vi "read_db_for_file_relocation.vi"(7 "Small?":bool, 8 "error in (no error)":errorcluster, 11 "File Location":T1=-2 items=["Unknown"=-5, "IDL Processing"=-4, "Writing from Queue"=-3, "Labview Files"=-2, "Retry Labview files"=-1, "Local Cache "=0, "Storage"=1]) -> (0 "error out":errorcluster, 3 "BP Array":T2[](array[typedef]) {"File Location" items=["Unknown"=-5, "IDL Processing"=-4, "Writing from Queue"=-3, "Labview Files"=-2, "Retry Labview files"=-1, "Local Cache "=0, "Storage"=1]})   [LabVIEW 2013]
uses:
  Batch Processor/bp_cluster.ctl
  Controls/File_location.ctl
  <vilib>/addons/database/Auxilliary.llb/DB Tools Parameter Info.ctl
  <vilib>/addons/database/Auxilliary.llb/DB Tools DataTypes.ctl
  <vilib>/addons/database/Auxilliary.llb/DB Tools Parameter Dir.ctl
  <vilib>/addons/database/Command.llb/Cmd Set Parameter Value (C).vi
  <vilib>/addons/database/Command.llb/Cmd Execute.vi
  <vilib>/addons/database/Recordset.llb/Rec Fetch Recordset Data (CR).vi
  <vilib>/addons/database/Recordset.llb/Rec Destroy - Command.vi
  <vilib>/addons/database/Command.llb/Cmd Delete.vi
  <vilib>/addons/database/_DB Variant To Data/Database Variant To Data.xnode
  <vilib>/addons/database/NI_Database_API.lvlib
panel:
  out "size(s)":i32
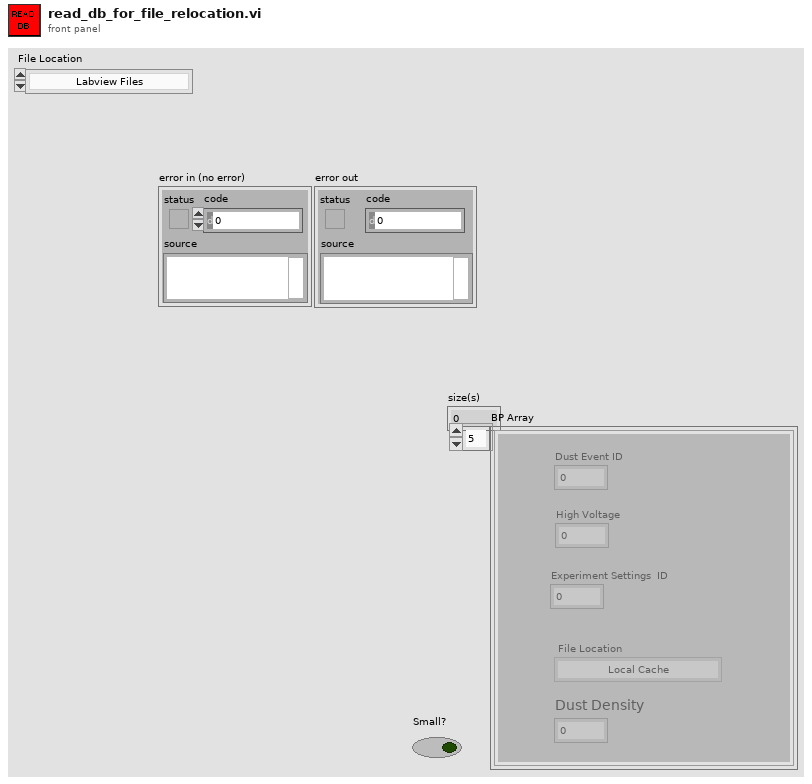
[diagram p1: front panel]
types:
  T1 = typedef "File_location.ctl" = i8
  T2 = typedef "bp_cluster.ctl" = cluster{"Dust Event ID":i64, "High Voltage":sgl, "Experiment Settings  ID":i64, "File Location":T1, "Dust Density":dbl}
  T3 = typedef "NI_Database_API.lvlib/DB Tools Parameter Info.ctl" = cluster{"parameter name":string, "type":T4, "direction":T5, "value":variant}
  T4 = typedef "NI_Database_API.lvlib/DB Tools DataTypes.ctl" = enum16{"String", "Long (I32)", "Single (SGL)", "Double (DBL)", "Date/Time", "Binary"}
  T5 = typedef "NI_Database_API.lvlib/DB Tools Parameter Dir.ctl" = enum32{"Input", "Output", "Input/Output", "Return Value"}
  T6 = typedef "NI_Database_API.lvlib/Conn ObjectReference.ctl" = refnum<k1>
  T7 = typedef "NI_Database_API.lvlib/Cmd ObjectReference.ctl" = refnum<k1>
  T8 = typedef "NI_Database_API.lvlib/Cmd-Rec Object Reference.ctl" = refnum<k1>
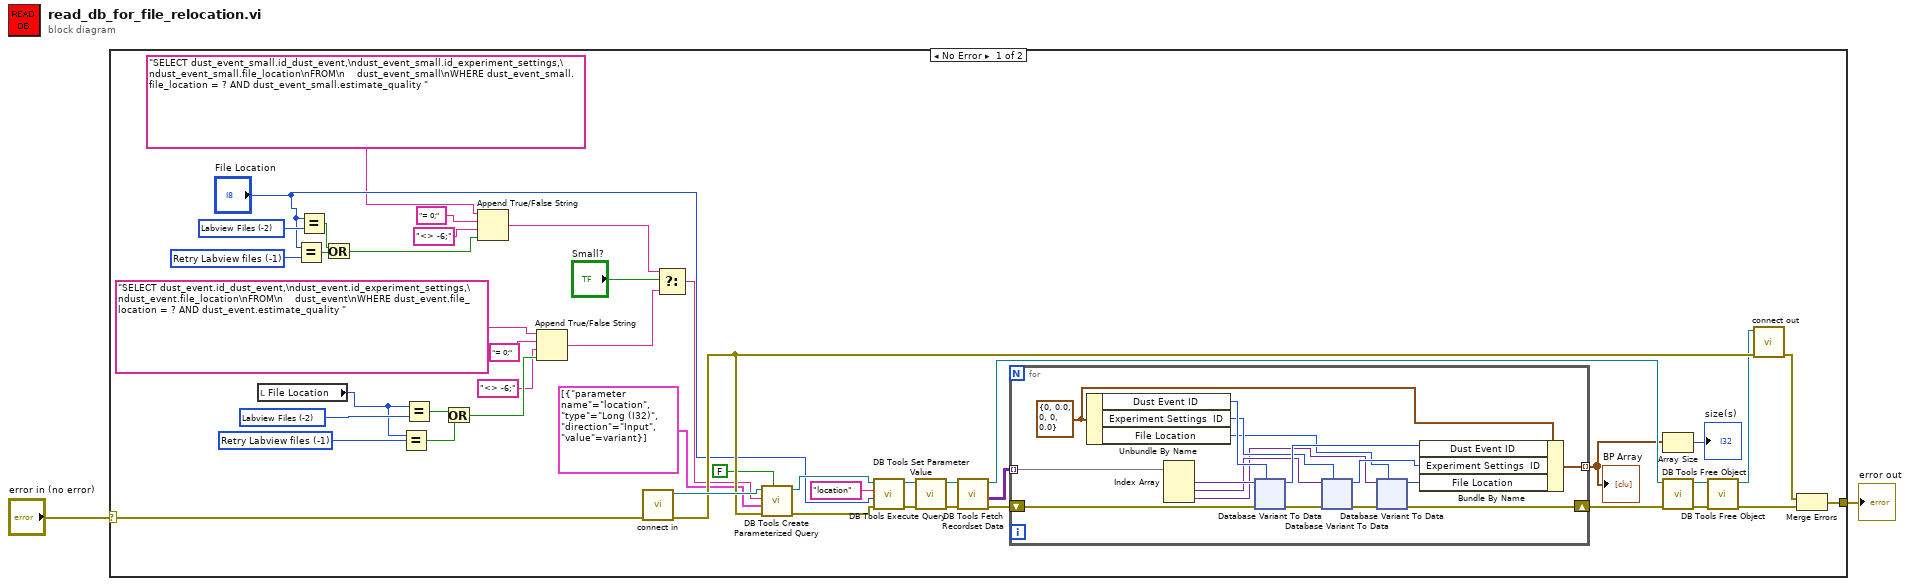
[diagram p0: block diagram]
diagram:
  n1 = case shown="No Error" "error in (no error)" {
    selector: "error in (no error)" -> [w26 w161]
    tunnel: [w37 w161] -> w1
    frame No Error {
      w14 = T1 -1 items=["Unknown"=-5, "IDL Processing"=-4, "Writing from Queue"=-3, "Labview Files"=-2, "Retry Labview files"=-1, "Local Cache "=0, "Old Storage"=1, "Storage"=2] ("y")
      w19 = T1 -2 items=["Labview Files"=-2, "Mars Data Processing Factility"=-1, "Local Cache "=0, "Old Storage"=1, "Storage"=2] ("y")
      w21 = T1 -1 items=["Unknown"=-5, "IDL Processing"=-4, "Writing from Queue"=-3, "Labview Files"=-2, "Retry Labview files"=-1, "Local Cache "=0, "Old Storage"=1, "Storage"=2] ("y")
      w40 = T1 -2 items=["Labview Files"=-2, "Mars Data Processing Factility"=-1, "Local Cache "=0, "Old Storage"=1, "Storage"=2] ("y")
      n2 = local read "File Location"() -> (w13:T1)
      n3 = Equal?(x="File Location", y=w21) -> (x = y?=w20:bool)
      n4 = Equal?(x="File Location", y=w40) -> (x = y?=w39:bool)
      n5 = Or(x=w39, y=w20) -> (x .or. y?=w9:bool)
      n6 = Equal?(x=w13, y=w14) -> (x = y?=w16:bool)
      n7 = Equal?(x=w13, y=w19) -> (x = y?=w15:bool)
      n8 = Or(x=w15, y=w16) -> (x .or. y?=w7:bool)
      n9 = Append True/False String(1:w9, 2:"<> -6;", 3:"= 0;", 4:"SELECT dust_event_small.id_dust_event,\ndust_event_small.id_experiment_settings,\ndust_event_small.file_location\nFROM\n    dust_event_small\nWHERE dust_event_small.file_location = ? AND dust_event_small.estimate_quality " ("string")) -> (0:w8:string)
      n10 = Append True/False String(1:w7, 2:"<> -6;", 3:"= 0;", 4:"SELECT dust_event.id_dust_event,\ndust_event.id_experiment_settings,\ndust_event.file_location\nFROM\n    dust_event\nWHERE dust_event.file_location = ? AND dust_event.estimate_quality " ("string")) -> (0:w3:string)
      n11 = call "connect in.vi"("error in (no error)"=w26) -> ("error out"=w35:errorcluster, "Database Connection"=w36:T6)  [unwired: 6 in, 1 out]
      n12 = Select(t=w8, s="Small?", f=w3) -> (s? t:f=w18:string)
      n13 = call <vilib>:"DB Tools Create Parameterized Query.vi"("auto-detect parameters? (F)"=FALSE, "error in (no error)"=w35, "parameters"=T3[] [{"parameter name"="location", "type"=enum."Long (I32)", "direction"=enum."Input", "value"=variant}], "SQL query"=w18, "connection reference"=w36) -> ("error out"=w33:errorcluster, "command reference"=w34:T7)  [unwired: 2 in, 1 out]
      n14 = call-poly <vilib>:"DB Tools Set Parameter Value.vi"("error in (no error)"=w33, "value"="File Location", "parameter index"="location" ("parameter name"), "command reference"=w34) -> ("error out"=w27:errorcluster, "command reference out"=w28:T7)  [unwired: 4 in]
      n15 = call-poly <vilib>:"DB Tools Execute Query.vi"("error in (no error)"=w27, "command reference"=w28) -> ("error out"=w47:errorcluster, "command-recordset reference"=w48:T8)  [unwired: 6 in]
      n16 = call-poly <vilib>:"DB Tools Fetch Recordset Data.vi"("error in (no error)"=w47, "command-recordset reference"=w48) -> ("error out"=w45:errorcluster, "recordset data"=w43:variant[][], "command-recordset reference out"=w46:T8)  [unwired: 3 in]
      n17 = for {
        tunnel: w43 -> [w64] mode=indexing
        shift-right: [w49] -> w44
        shift-left: w45 -> [w63]
        tunnel: [w61] -> w42 mode=indexing
        w58 = T2 {"Dust Event ID"=0, "High Voltage"=0.0, "Experiment Settings  ID"=0, "File Location"=0, "Dust Density"=0.0} ("Batch Processing Cluster")
        n18 = Unbundle By Name(w58) -> ("Dust Event ID"=w60:i64, "Experiment Settings  ID"=w57:i64, "File Location"=w52:T1)
        n19 = Index Array(array=w64) -> (element #1=w62:variant, element #2=w54:variant, element #3=w53:variant)  [unwired: 3 in]
        n20 = xnode "Database Variant To Data"("database variant"=w62, "error in"=w63, "type"=w60) -> ("data"=w59:i64, "error out"=w55:errorcluster)
        n21 = xnode "Database Variant To Data"("database variant"=w54, "error in"=w55, "type"=w57) -> ("data"=w56:i64, "error out"=w50:errorcluster)
        n22 = xnode "Database Variant To Data"("database variant"=w53, "error in (no error)"=w50, "type"=w52) -> ("data"=w51:T1, "error out"=w49:errorcluster)
        n23 = Bundle By Name(cluster=w58, "Dust Event ID"=w59, "Experiment Settings  ID"=w56, "File Location"=w51) -> (w61:T2)
      }
      "BP Array" <- w42
      n24 = Array Size(array=w42) -> (size(s)=→"size(s)":i32)
      n25 = call-poly <vilib>:"DB Tools Free Object.vi"("error in (no error)"=w44, "command-recordset reference"=w46) -> ("error out"=w31:errorcluster, "command reference"=w23:T7)  [unwired: 8 in]
      n26 = call-poly <vilib>:"DB Tools Free Object.vi"("error in (no error)"=w31, "command reference"=w23) -> ("error out"=w30:errorcluster, "connection reference"=w32:T6)  [unwired: 8 in]
      n27 = call "connect out.vi"("error in (no error)"=w35, "connection reference"=w32) -> ("error out"=w38:errorcluster)  [unwired: 9 in]
      n28 = Merge Errors(w38, w30) -> (w37:errorcluster)
    }
    frame Error {
    }
  }
  "error out" <- w1
